vi "Get VIPM Dependency Map.vi"(7 "Force Reload?(F)":bool, 8 "error in":errorcluster) -> (0 "error out":errorcluster, 1 "Unmatched Packages":string[](array[string]), 2 "Internal Target Map":map{string, string}(c390), 3 "Package Array":T1[](array[typedef]))   [LabVIEW 2019, in "Project.Dependencies Finder.lvlib" / "Dependency Source_VIPM.lvclass"]
doc: "Get paths related to all known packages and return them in a map matching them to the package name.\n\n2020-11-11: Henrik Dueholm Hansen"
uses:
  Dependency Source_VIPM.lvclass
  Ctl/Ctl_Package Identifier Cluster.ctl
  ce6ecaaf-38ea-4476-9fc5-063443edb655.vi
  <vilib>/Utility/config.llb/NI_LVConfig.lvlib
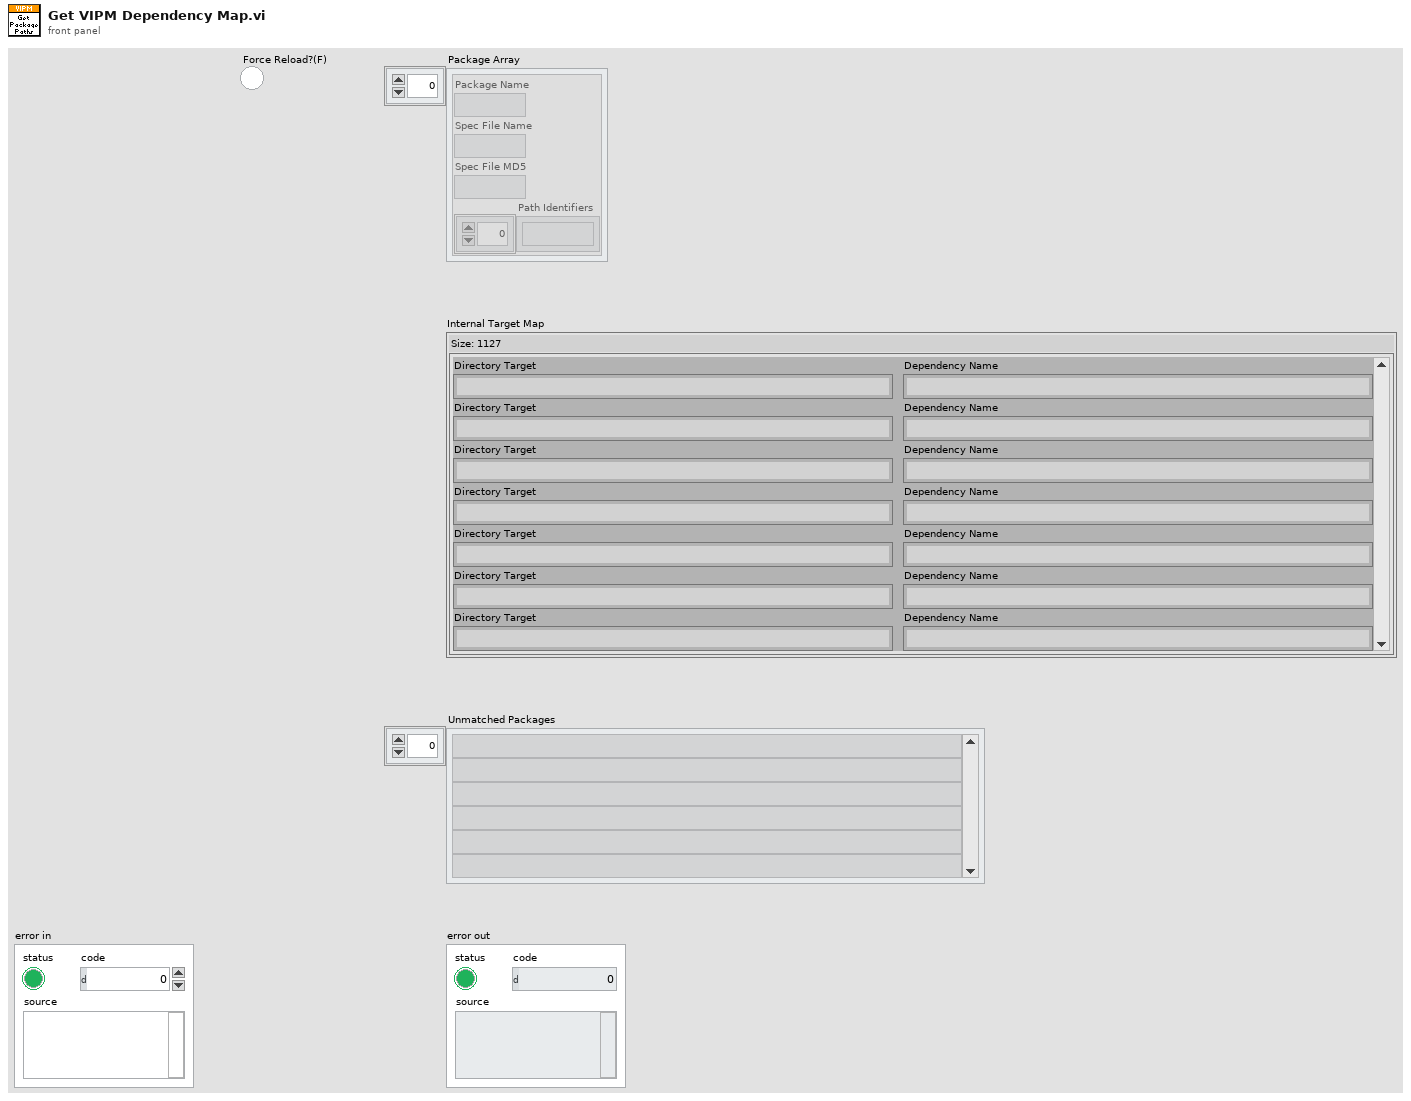
[diagram p1: front panel]
types:
  T1 = typedef "Project.Dependencies Finder.lvlib/Dependency Source_VIPM.lvclass/Ctl_Package Identifier Cluster.ctl" = cluster{"Package Name":string, "Spec File Name":string, "Spec File MD5":string, "Path Identifiers":string[]}
  T2 = typedef "NI_LVConfig.lvlib/Config Data RefNum.ctl" = refnum<k1>
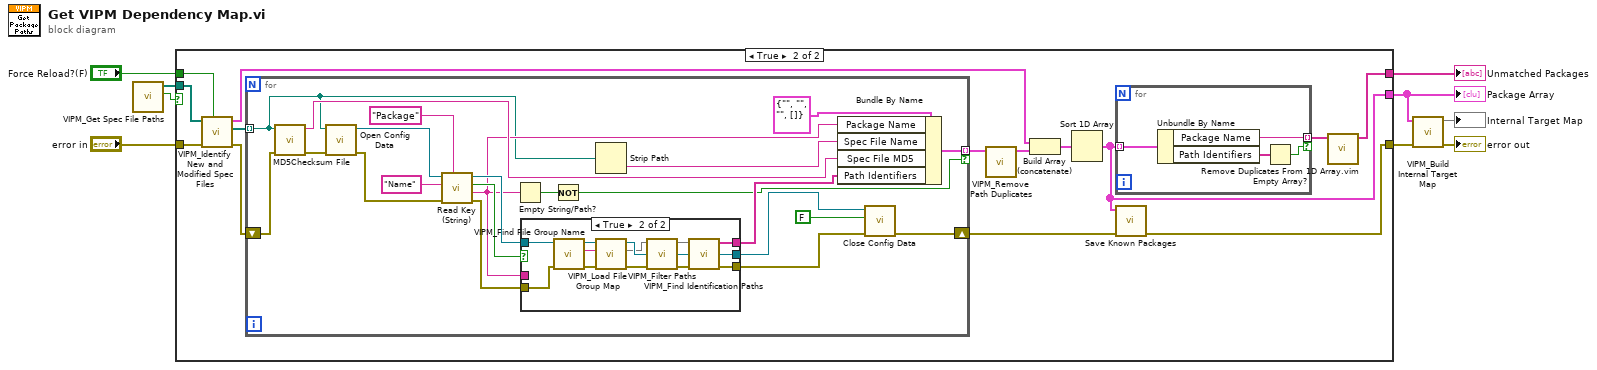
[diagram p0: block diagram]
diagram:
  n1 = call "VIPM_Get Spec File Paths.vi"() -> ("Success?"=w3:bool, "Spec Paths"=w6:path[])  [unwired: 10 in]
  n2 = case shown="True" w3 {
    tunnel: [w9 w13] -> w7
    tunnel: "error in" -> [w9 w16]
    tunnel: w6 -> [_ w21]
    tunnel: [_ w10] -> w5
    tunnel: [_ w15] -> w4
    tunnel: "Force Reload?(F)" -> [_ w12]
    frame False {
    }
    frame True {
      n3 = call "VIPM_Identify New and Modified Spec Files.vi"("Force Reload?(F)"=w12, "error in (no error)"=w16, "Spec Files"=w21) -> ("error out"=w17:errorcluster, "New or Modified Spec Files"=w20:path[], "Unchanged Package Array"=w18:T1[])  [unwired: 6 in]
      n4 = for {
        shift-right: [w32] -> w14
        shift-left: w17 -> [w31]
        tunnel: [w36] -> w23 mode=indexing if=w33
        tunnel: w20 -> [w29] mode=indexing
        n5 = call <vilib>:"MD5Checksum File.vi"("error in (no error)"=w31, "Path"=w29) -> ("error out"=w30:errorcluster, "MD5 message-digest"=w38:string)  [unwired: 8 in]
        n6 = call <vilib>:"Open Config Data.vi"("error in (no error)"=w30, "configuration file path"=w29) -> ("error out"=w45:errorcluster, "refnum"=w49:T2)  [unwired: 7 in, 1 out]
        n7 = call <vilib>:"Read Key (String).vi"("section"="Package", "error in (no error)"=w45, "key"="Name", "refnum"=w49) -> ("error out"=w40:errorcluster, "value"=w35:string, "found?"=w46:bool, "refnum out"=w44:T2)  [unwired: 4 in]
        n8 = Empty String/Path?(string/path=w35) -> (empty?=w34:bool)
        n9 = case shown="True" w46 {
          tunnel: w44 -> [w51 w61]
          tunnel: [w51 w57] -> w43
          tunnel: [w50 w56] -> w41
          tunnel: w40 -> [w50 w60]
          tunnel: w35 -> [_ _]
          tunnel: [_ w52] -> w37
          frame False {
          }
          frame True {
            n10 = call "VIPM_Find File Group Name.vi"("error in (no error)"=w60, "Refnum in"=w61) -> ("error out"=w58:errorcluster, "File Group Name"=w55:string, "Refnum out"=w59:T2)  [unwired: 7 in]
            n11 = call "VIPM_Load File Group Map.vi"("error in (no error)"=w58, "File Group Name"=w55, "Refnum in"=w59) -> ("error out"=w56:errorcluster, "Ordered File Group map"=w53:map{string, string[]}, "Refnum out"=w57:T2)  [unwired: 6 in]
            n12 = call "VIPM_Filter Paths.vi"("Unfiltered map in"=w53) -> ("Filtered map out"=w54:map{string, string[]})  [unwired: 10 in]
            n13 = call "VIPM_Find Identification Paths.vi"("Filtered map in"=w54) -> ("Found Identification Paths"=w52:string[])  [unwired: 10 in]
          }
        }
        n14 = Not(x=w34) -> (.not. x?=w33:bool)
        n15 = Strip Path(path=w29) -> (name=w28:string)  [unwired: 1 out]
        n16 = Bundle By Name(cluster=T1 {"Package Name"="", "Spec File Name"="", "Spec File MD5"="", "Path Identifiers"=[]}, "Package Name"=w35, "Spec File Name"=w28, "Spec File MD5"=w38, "Path Identifiers"=w37) -> (w36:T1)
        n17 = call <vilib>:"Close Config Data.vi"("error in (no error)"=w41, "write file if changed (T)"=FALSE, "refnum"=w43) -> ("error out"=w32:errorcluster)  [unwired: 7 in, 1 out]
      }
      n18 = call "VIPM_Remove Path Duplicates.vi"("Package Array in"=w23) -> ("Package Array out"=w22:T1[])  [unwired: 10 in]
      n19 = Build Array (concatenate)(w18, w22) -> (w19:T1[])
      n20 = Sort 1D Array(array=w19) -> (sorted array=w15:T1[])
      n21 = for {
        tunnel: w15 -> [w27] mode=indexing
        tunnel: [w25] -> w11 mode=indexing if=w24
        n22 = Unbundle By Name(w27) -> ("Package Name"=w25:string, "Path Identifiers"=w26:string[])
        n23 = Empty Array?(array=w26) -> (empty?=w24:bool)
      }
      n24 = call "Save Known Packages.vi"("error in (no error)"=w14, "Package Array from File"=w15) -> ("error out"=w13:errorcluster)  [unwired: 8 in, 1 out]
      n25 = call "Remove Duplicates From 1D Array.vim"("array"=w11) -> ("array with duplicates removed"=w10:string[])  [unwired: 10 in]
    }
  }
  "error out" <- w7
  "Unmatched Packages" <- w5
  "Package Array" <- w4
  n26 = call "VIPM_Build Internal Target Map.vi"("Package Array"=w4) -> ("Internal Target Map"=→"Internal Target Map":map{string, string})  [unwired: 10 in]
